vi "ObserverInit.vi"() -> ()   [LabVIEW 2018]
uses:
  D:/Elt/Framework2.1/variantlib_code/Abstract_Actor/Abstract_Actor/Abstract_Actor.lvclass
  D:/Elt/Framework2.1/variantlib_code/Abstract_Actor/Abstract_Actor/Abstract_Actor.lvclass/Abstract_Actor.ctl
  D:/Elt/Framework2.1/variantlib/General_Support.lvlibp
  <vilib>/Utility/Data Type/NI_Data Type.lvlib
panel:
  out "Element_Name":string[](array[string])
  out "observedDataChanged":bool[](array[boolean])
  out "Cluster_out":variant[](array[variant])
  out "allActorDataName":string[](array[string])
  out "actorDataChanged":bool
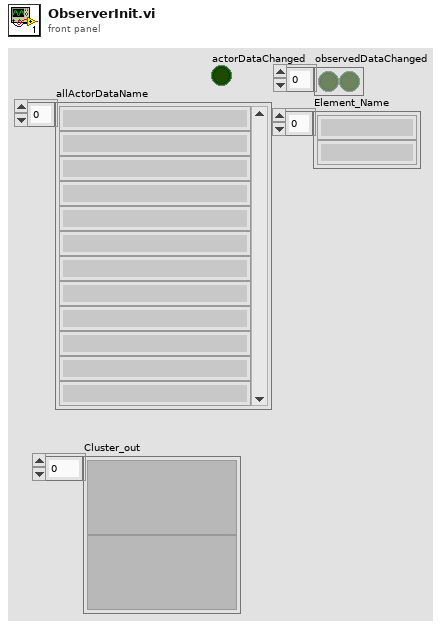
[diagram p1: front panel]
types:
  T1 = cluster{"Caller_Alias":string, "Actor_Alias":string}
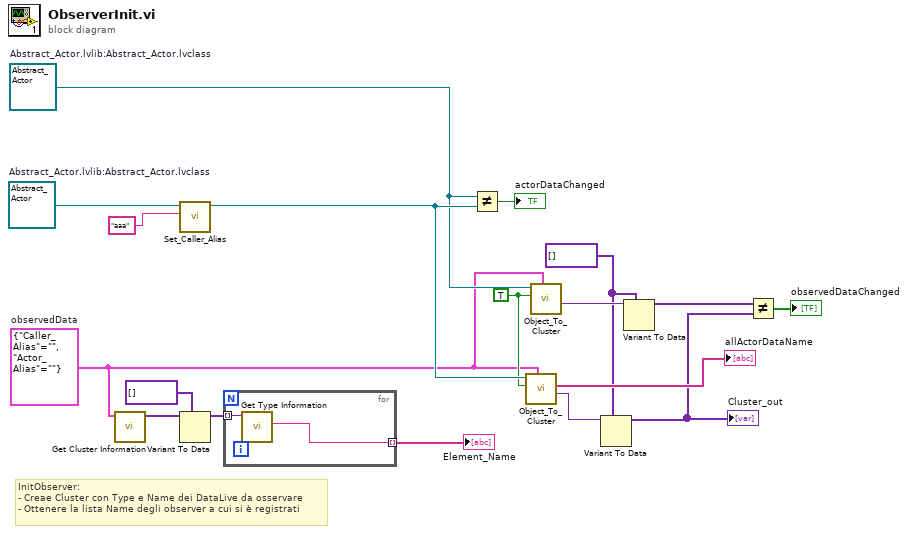
[diagram p0: block diagram]
diagram:
  w7 = TRUE ("All_Hierarchy (F)")
  w10 = variant[] [] ("type")
  w5 = T1 {"Caller_Alias"="", "Actor_Alias"=""}  # observedData
  w17 = refnum<class "Abstract_Actor.lvclass"> refnum  # Abstract_Actor.lvlib:Abstract_Actor.lvclass
  w6 = refnum<class "Abstract_Actor.lvclass"> refnum  # Abstract_Actor.lvlib:Abstract_Actor.lvclass
  # "InitObserver:\n- Creae Cluster con Type e Name dei DataLive da osservare\n- Ottenere la lista Name degli observer a cui si è registrati"
  n1 = call <vilib>:"Get Cluster Information.vi"("Variant"=w5) -> ("Cluster Elements"=w4:variant[])  [unwired: 9 in, 1 out]
  n2 = call "Set_Caller_Alias.vi"("Caller_Alias"="aaa", "Abstract_Actor in"=w17) -> ("Abstract_Actor out"=w15:refnum<class "Abstract_Actor.lvclass">)  [unwired: 8 in, 1 out]
  n3 = Variant To Data(type=variant[] [], Variant=w4) -> (data=w2:variant[])  [unwired: 1 in, 1 out]
  n4 = for {
    tunnel: w2 -> [w20] mode=indexing
    tunnel: [w19] -> w1 mode=indexing
    n5 = call <vilib>:"Get Type Information.vi"("Variant"=w20) -> ("Name"=w19:string)  [unwired: 6 in, 4 out]
  }
  "Element_Name" <- w1
  n6 = Not Equal?(x=w6, y=w15) -> (x != y?=→"actorDataChanged":bool)
  n7 = call "Object_To_Cluster.vi"("Cluster_Type"=w5, "All_Hierarchy (F)"=w7, "LabVIEW_Object"=w15) -> ("Cluster_out"=w11:variant, "Element_Name"=→"allActorDataName":string[])  [unwired: 5 in, 2 out]
  n8 = call "Object_To_Cluster.vi"("Cluster_Type"=w5, "All_Hierarchy (F)"=w7, "LabVIEW_Object"=w6) -> ("Cluster_out"=w13:variant)  [unwired: 5 in, 3 out]
  n9 = Variant To Data(type=w10, Variant=w11) -> (data=w9:variant[])  [unwired: 1 in, 1 out]
  "Cluster_out" <- w9
  n10 = Variant To Data(type=w10, Variant=w13) -> (data=w12:variant[])  [unwired: 1 in, 1 out]
  n11 = Not Equal?(x=w12, y=w9) -> (x != y?=→"observedDataChanged":bool[])
